vi "用户列表.vi"() -> ()   [LabVIEW 2016, in "Alarm interface.lvlib" / "wxpusher.lvlib"]
uses:
  wxpusher.lvlib
  <vilib>/Utility/miscctls.llb/LVPointTypeDef.ctl
panel:
  in  "关闭":bool
  in  "删除":bool
  in  "添加":bool
  in  "微信用户列表":i32(listbox)
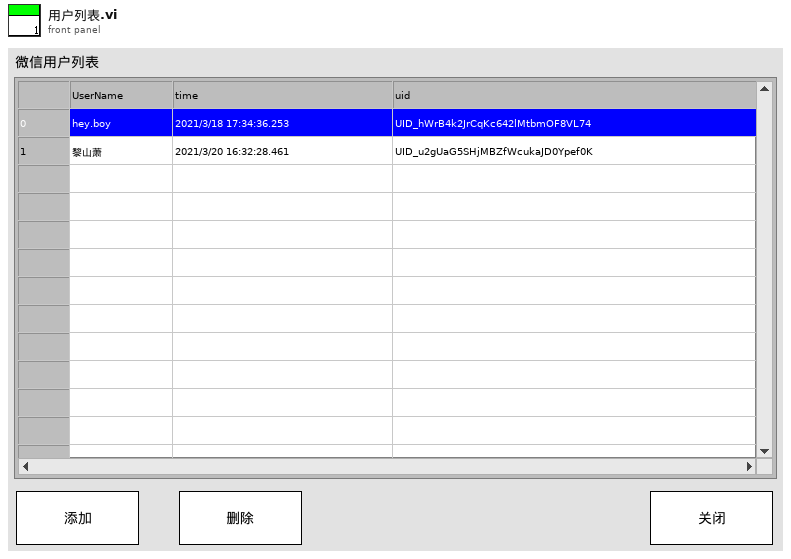
[diagram p1: front panel]
types:
  T1 = typedef "LVPointTypeDef.ctl" = cluster{"Horizontal":i16, "Vertical":i16}
  T2 = cluster{"action":string, "data":cluster{"appKey":string, "appName":string, "source":string, "time":u64, "uid":string, "userHeadImg":string, "userName":string, "extra":string}}[]
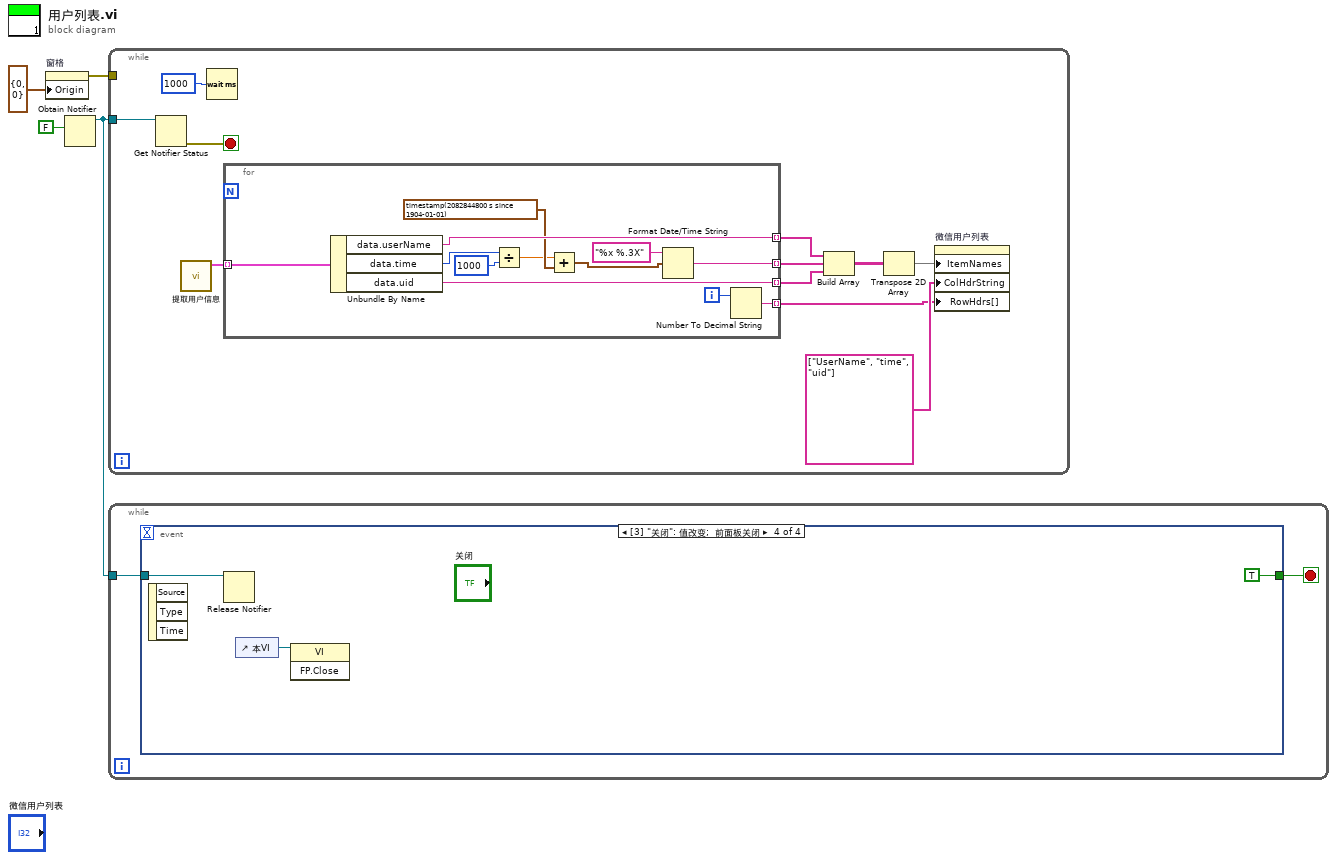
[diagram p0: block diagram]
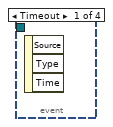
[diagram p2: hidden frame]
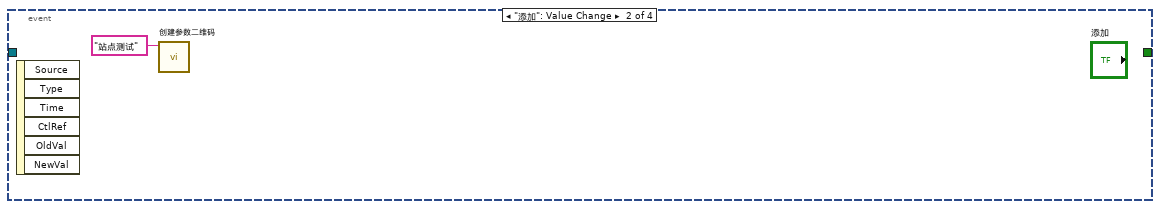
[diagram p3: hidden frame]
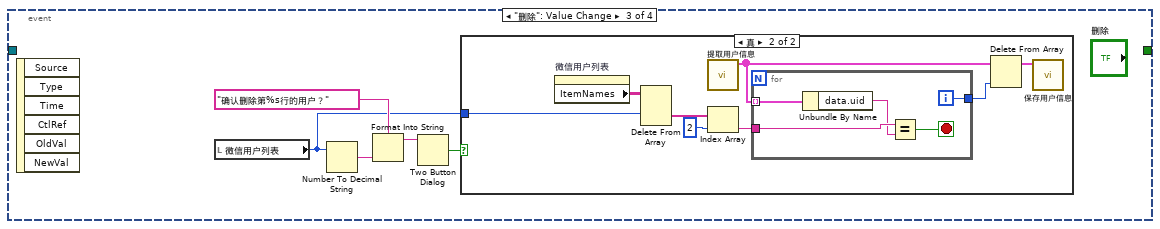
[diagram p4: hidden frame]
diagram:
  n1 = property on="窗格" class="Pane"("Origin"=T1 {"Horizontal"=0, "Vertical"=0} ("原点")) -> (error out=w3:errorcluster)  [unwired: 2 in, 1 out]
  n2 = Obtain Notifier(notification data type=FALSE) -> (notifier out=w1:refnum<notifier>)  [unwired: 3 in, 2 out]
  n3 = while {
    tunnel: w3 -> [_]
    tunnel: w1 -> [w6]
    stop <- w5 stop-if-true
    n4 = Get Notifier Status(notifier=w6) -> (error out=w5:errorcluster)  [unwired: 1 in, 4 out]
    n5 = call "提取用户信息.vi"() -> ("用户信息"=w15:T2)  [unwired: 10 in, 1 out]
    n6 = Wait (ms)(milliseconds to wait=u32 1000 ("等待时间（毫秒）")) -> ()  [unwired: 1 out]
    n7 = for {
      tunnel: w15 -> [w27] mode=indexing
      tunnel: [w26] -> w14 mode=indexing
      tunnel: [w25] -> w12 mode=indexing
      tunnel: [w18] -> w13 mode=indexing
      tunnel: [w16] -> w7 mode=indexing
      i -> [w17]
      n8 = Unbundle By Name(w27) -> ("data.userName"=w26:string, "data.time"=w19:u64, "data.uid"=w25:string)
      n9 = Divide(x=w19, y=u64 1000) -> (x/y=w21:dbl)
      n10 = Add(x=w21, y=timestamp(2082844800 s since 1904-01-01)) -> (x+y=w23:timestamp)
      n11 = Format Date/Time String(time format string (%c)="%x %.3X" ("时间格式字符串(%c)"), seconds (now)=w23) -> (date/time string=w18:string)  [unwired: 1 in]
      n12 = Number To Decimal String(number=w17) -> (decimal integer string=w16:string)  [unwired: 1 in]
    }
    n13 = Build Array(w14, w13, w12) -> (w11:string[][])
    n14 = Transpose 2D Array(2D array=w11) -> (transposed array=w10:string[][])
    n15 = property on="微信用户列表" class="MCListbox (严格)"("ItemNames"=w10, "ColHdrString"=string[] ["UserName", "time", "uid"] ("列首字符串[]"), "RowHdrs[]"=w7) -> ()  [unwired: 2 in, 2 out]
  }
  n16 = while {
    tunnel: w1 -> [w28]
    stop <- w29 stop-if-true
    n17 = event shown="[3] \"关闭\": 值改变;  前面板关闭" {
      selector: _ -> [_ _ _ _]
      dyn-events: _ -> [_ _ _ _]
      timeout: _ -> [_ _ _ _]
      tunnel: [_ _ _ TRUE] -> w29
      tunnel: w28 -> [_ _ _ w49]
      event Timeout {
        n18 = event-data() -> ()  [unwired: 1 in, 3 out]
      }
      event "添加": Value Change {
        n19 = event-data() -> ()  [unwired: 1 in, 6 out]
        n20 = call "创建参数二维码.vi"("站点"="站点测试") -> ()  [unwired: 11 in]
      }
      event "删除": Value Change {
        n21 = event-data() -> ()  [unwired: 1 in, 6 out]
        n22 = local read "微信用户列表"() -> (w34:i32)
        n23 = Number To Decimal String(number=w34) -> (decimal integer string=w33:string)  [unwired: 1 in]
        n24 = Format Into String(format string="确认删除第%s行的用户？" ("消息"), w33) -> (resulting string=w32:string)  [unwired: 2 in, 1 out]
        n25 = Two Button Dialog(message=w32) -> (T button?=w31:bool)  [unwired: 2 in]
        n26 = case shown="真" w31 {
          tunnel: w34 -> [_ w42]
          frame False {
          }
          frame True {
            n27 = property on="微信用户列表" class="MCListbox (严格)"() -> ("ItemNames"=w43:string[][])  [unwired: 2 in, 2 out]
            n28 = Delete From Array(array=w43, index (row)=w42) -> (deleted portion=w41:string[])  [unwired: 2 in, 1 out]
            n29 = call "提取用户信息.vi"() -> ("用户信息"=w38:T2)  [unwired: 10 in, 1 out]
            n30 = Index Array(array=w41, index=2 ("索引")) -> (element=w39:string)
            n31 = for {
              tunnel: w38 -> [w48] mode=indexing
              tunnel: w39 -> [w47]
              tunnel: [w44] -> w37
              i -> [w44]
              stop <- w45 stop-if-true
              n32 = Unbundle By Name(w48) -> ("data.uid"=w46:string)
              n33 = Equal?(x=w47, y=w46) -> (x = y?=w45:bool)
            }
            n34 = Delete From Array(array=w38, index=w37) -> (array with subset deleted=w36:T2)  [unwired: 1 in, 1 out]
            n35 = call "保存用户信息.vi"("用户信息"=w36) -> ()  [unwired: 10 in, 1 out]
          }
        }
      }
      event "关闭": Value Change; Panel Close {
        n36 = event-data() -> ()  [unwired: 1 in, 3 out]
        n37 = Release Notifier(notifier=w49) -> ()  [unwired: 2 in, 3 out]
        n38 = control-ref of="本VI"() -> (w51:refnum<vi>)
        n39 = invoke class="VI" method="FP.Close"(reference=w51) -> ()  [unwired: 2 in, 3 out]
      }
    }
  }
